vi "StateShooter.vi"(1 "Master State":enum16{"Normal", "Climb"}(ring)) -> (0 "Shooter Firing":bool)   [LabVIEW 2020]
doc: "Performs all of the calculations and decisions related to the shooter including the cowl positon."
uses:
  3e13d083-b44f-41ac-8210-6ef27915361f.vi
  31b76865-9f3e-4ec7-bf23-6a72130b3556.vi
  drivercommands.vi
  robotoutputs.vi
  robotconstants.vi
  driverdata.vi
  autonomousinfo.vi
  sensordata.vi
panel:
  in  "Max Robot Velocity Change (ft/s)":dbl=0.5
  in  "Kicker Goal Speed (rpm)":dbl=3000.0
  in  "Acceptable Kicker Error (rpm)":dbl=150.0
  in  "Acceptable Upper Shooter Error (rpm)":dbl=250.0
  in  "Minimum Range (in)":dbl=50.0
  in  "Maximum Range (in)":dbl=300.0
  in  "Acceptable Cowl Error (deg)":dbl=1.0
  in  "Acceptable Lower Shooter Error (rpm)":dbl=150.0
  in  "Settling Time (ms)":u32=100
  in  "Shooter Prespin (ms)":u32=30000
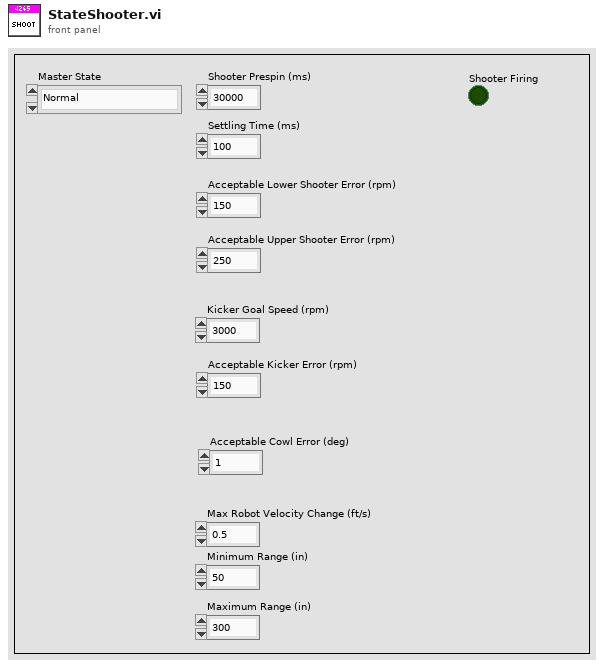
[diagram p1: front panel]
types:
  T1 = enum16{"Targetting Computer", "Position 1", "Position 2", "Position 3", "Position 4"}
  T2 = typedef "WPI_DriverStationAllianceInfo.ctl" = enum16{"Red", "Blue", "Invalid"}
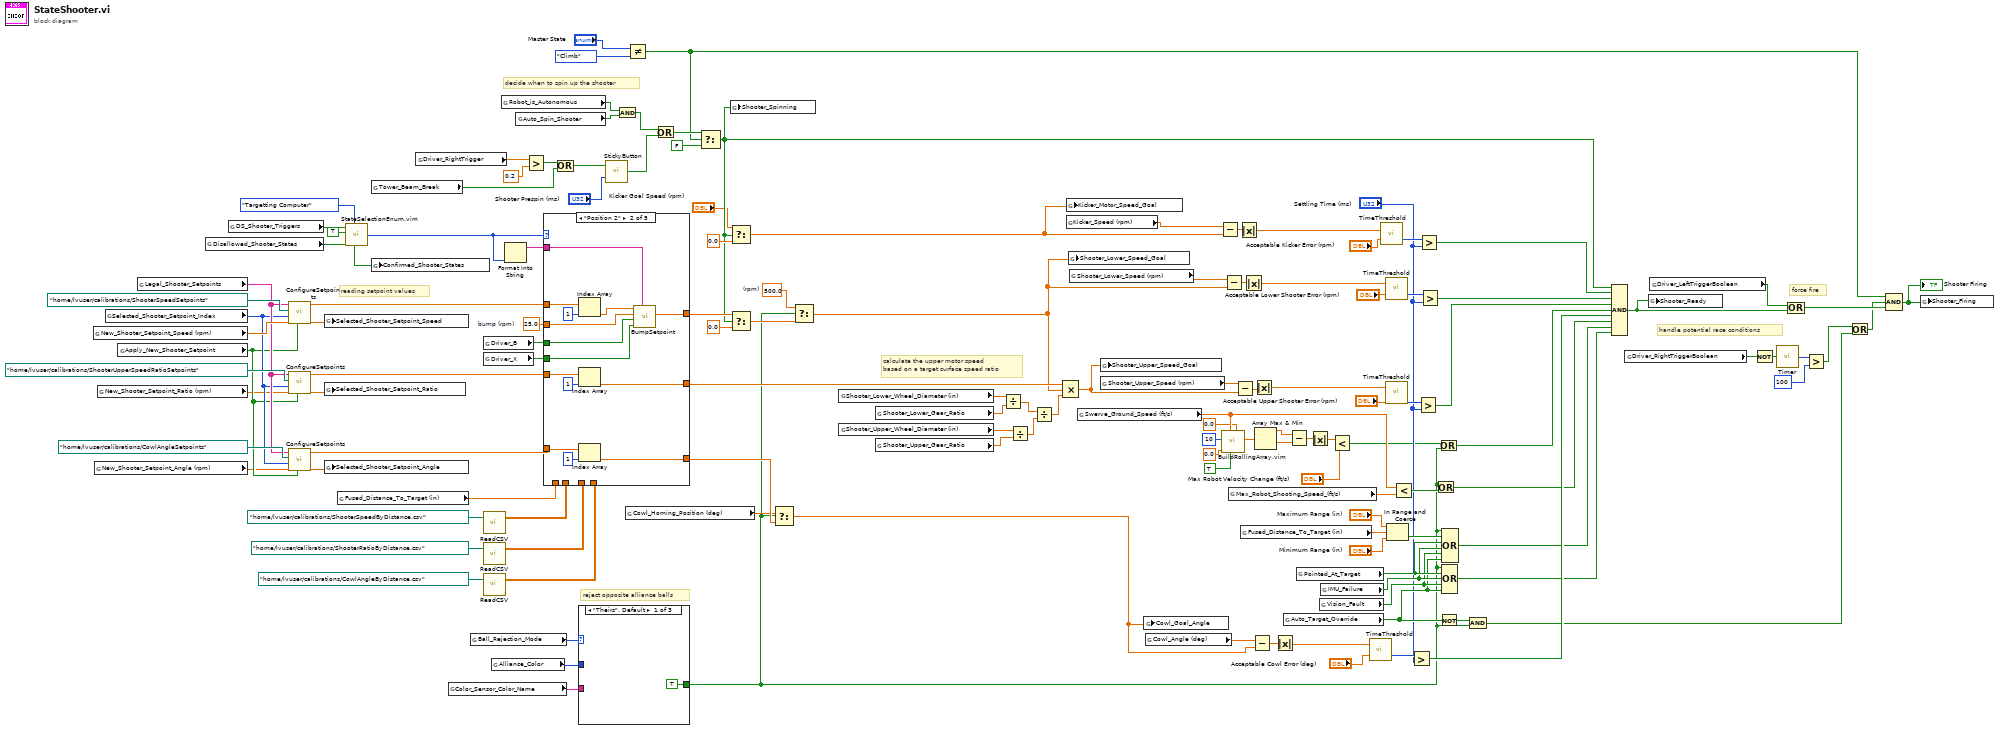
[diagram p0: block diagram]
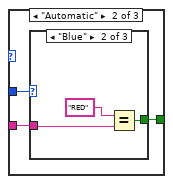
[diagram p2: hidden frame]
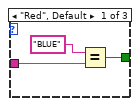
[diagram p3: hidden frame]
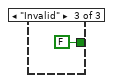
[diagram p4: hidden frame]
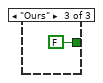
[diagram p5: hidden frame]
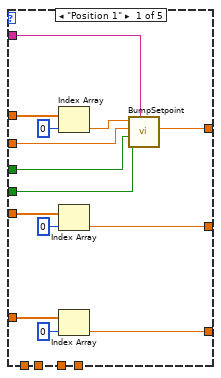
[diagram p6: hidden frame]
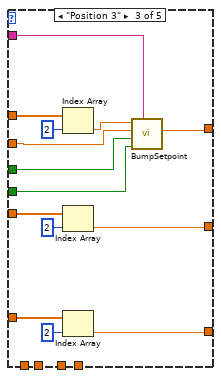
[diagram p7: hidden frame]
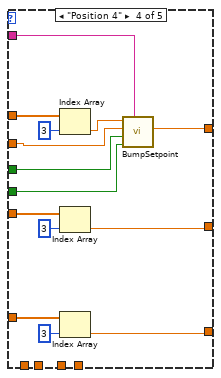
[diagram p8: hidden frame]
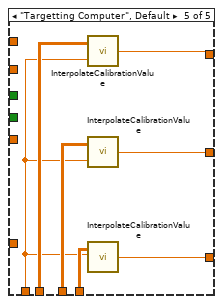
[diagram p9: hidden frame]
diagram:
  w1 = 500.0  # (rpm)
  w84 = 25.0  # bump (rpm)
  # "handle potential race conditions"
  # "calculate the upper motor speed\nbased on a target surface speed ratio"
  # "reject opposite alliance balls"
  # "force fire"
  # "reading setpoint values"
  # "decide when to spin up the shooter"
  n1 = global read "driverdata.vi" "New_Shooter_Setpoint_Speed (rpm)"() -> (w129:dbl)
  n2 = global read "driverdata.vi" "New_Shooter_Setpoint_Angle (rpm)"() -> (w119:dbl)
  n3 = global read "driverdata.vi" "New_Shooter_Setpoint_Ratio (rpm)"() -> (w120:dbl)
  n4 = global read "driverdata.vi" "Selected_Shooter_Setpoint_Index"() -> (w123:i32)
  n5 = global read "driverdata.vi" "Apply_New_Shooter_Setpoint"() -> (w121:bool)
  n6 = global read "robotconstants.vi" "Legal_Shooter_Setpoints"() -> (w124:string[])
  n7 = global read "robotoutputs.vi" "Disallowed_Shooter_States"() -> (w133:bool[])
  n8 = global read "drivercommands.vi" "DS_Shooter_Triggers"() -> (w135:bool[])
  n9 = call "ConfigureSetpoints.vi"("Apply New Setpoint"=w121, "New Setpoint"=w129, "Selected Setpoint Index"=w123, "Setpoint Save Location"=path "/home/lvuser/calibrations/ShooterSpeedSetpoints", "Setpoint Names"=w124) -> ("Selected Setpoint Value"=w118:dbl, "Setpoints"=w128:dbl[])  [unwired: 5 in]
  n10 = call "ConfigureSetpoints.vi"("Apply New Setpoint"=w121, "New Setpoint"=w120, "Selected Setpoint Index"=w123, "Setpoint Save Location"=path "/home/lvuser/calibrations/ShooterUpperSpeedRatioSetpoints", "Setpoint Names"=w124) -> ("Selected Setpoint Value"=w117:dbl, "Setpoints"=w126:dbl[])  [unwired: 5 in]
  n11 = call "ConfigureSetpoints.vi"("Apply New Setpoint"=w121, "New Setpoint"=w119, "Selected Setpoint Index"=w123, "Setpoint Save Location"=path "/home/lvuser/calibrations/CowlAngleSetpoints", "Setpoint Names"=w124) -> ("Selected Setpoint Value"=w116:dbl, "Setpoints"=w122:dbl[])  [unwired: 5 in]
  n12 = global write "robotoutputs.vi" "Selected_Shooter_Setpoint_Speed"(w118) -> ()
  n13 = global write "robotoutputs.vi" "Selected_Shooter_Setpoint_Ratio"(w117) -> ()
  n14 = global write "robotoutputs.vi" "Selected_Shooter_Setpoint_Angle"(w116) -> ()
  n15 = global read "sensordata.vi" "Fused_Distance_To_Target (in)"() -> (w87:dbl)
  n16 = call "StateSelectionEnum.vim"("Enum Def"=T1."Targetting Computer", "Disallowed States"=w133, "Enable Edge Trigger"=TRUE, "State Triggers"=w135) -> ("Selected State"=w81:T1, "Confirmed States"=w132:bool[])  [unwired: 1 in]
  n17 = global read "sensordata.vi" "Tower_Beam_Break"() -> (w41:bool)
  n18 = global write "robotoutputs.vi" "Confirmed_Shooter_States"(w132) -> ()
  n19 = global read "drivercommands.vi" "Driver_RightTrigger"() -> (w113:dbl)
  n20 = global read "sensordata.vi" "Color_Sensor_Color_Name"() -> (w64:string)
  n21 = global read "driverdata.vi" "Ball_Rejection_Mode"() -> (w61:enum16{"Theirs", "Automatic", "Ours"})
  n22 = call "ReadCSV.vi"("File Path (.csv)"=path "/home/lvuser/calibrations/ShooterSpeedByDistance.csv" ("Setpoint Save Location")) -> ("Data (index by row)"=w88:dbl[][])  [unwired: 1 in, 1 out]
  n23 = call "ReadCSV.vi"("File Path (.csv)"=path "/home/lvuser/calibrations/ShooterRatioByDistance.csv" ("Setpoint Save Location")) -> ("Data (index by row)"=w86:dbl[][])  [unwired: 1 in, 1 out]
  n24 = call "ReadCSV.vi"("File Path (.csv)"=path "/home/lvuser/calibrations/CowlAngleByDistance.csv" ("Setpoint Save Location")) -> ("Data (index by row)"=w85:dbl[][])  [unwired: 1 in, 1 out]
  n25 = global read "drivercommands.vi" "Driver_B"() -> (w83:bool)
  n26 = global read "drivercommands.vi" "Driver_X"() -> (w82:bool)
  n27 = global read "driverdata.vi" "Alliance_Color"() -> (w65:T2)
  n28 = global read "driverdata.vi" "Robot_is_Autonomous"() -> (w106:bool)
  n29 = Format Into String(w81) -> (resulting string=w80:string)  [unwired: 3 in, 1 out]
  n30 = global read "autonomousinfo.vi" "Auto_Spin_Shooter"() -> (w107:bool)
  n31 = Greater?(x=w113, y=0.2) -> (0:w111:bool)
  n32 = case shown="\"Position 2\"" w81 {
    tunnel: w128 -> [w149 w160 w174 w188 _]
    tunnel: w126 -> [w146 w159 w173 w187 _]
    tunnel: w122 -> [w143 w158 w172 w186 _]
    tunnel: [w137 w150 w168 w183 w197] -> w115
    tunnel: [w145 w157 w171 w185 w195] -> w45
    tunnel: [w142 w156 w170 w184 w192] -> w63
    tunnel: w88 -> [_ _ _ _ w198]
    tunnel: w87 -> [_ _ _ _ w193]
    tunnel: w86 -> [_ _ _ _ w196]
    tunnel: w85 -> [_ _ _ _ w194]
    tunnel: w84 -> [w140 w154 w166 w180 _]
    tunnel: w83 -> [w139 w153 w165 w179 _]
    tunnel: w82 -> [w138 w152 w164 w178 _]
    tunnel: w80 -> [w136 w151 w167 w181 _]
    frame "Position 1" {
      n33 = Index Array(array=w149, index=0) -> (element=w141:dbl)
      n34 = Index Array(array=w146, index=0) -> (element=w145:dbl)
      n35 = Index Array(array=w143, index=0) -> (element=w142:dbl)
      n36 = call "BumpSetpoint.vi"("Setpoint Name"=w136, "Bump Down Trigger"=w138, "Bump Up Trigger"=w139, "Bump Increment"=w140, "Original Setpoint"=w141) -> ("Bumped Setpoint"=w137:dbl)  [unwired: 6 in]
    }
    frame "Position 2" {
      n37 = Index Array(array=w160, index=1) -> (element=w155:dbl)
      n38 = Index Array(array=w159, index=1) -> (element=w157:dbl)
      n39 = Index Array(array=w158, index=1) -> (element=w156:dbl)
      n40 = call "BumpSetpoint.vi"("Setpoint Name"=w151, "Bump Down Trigger"=w152, "Bump Up Trigger"=w153, "Bump Increment"=w154, "Original Setpoint"=w155) -> ("Bumped Setpoint"=w150:dbl)  [unwired: 6 in]
    }
    frame "Position 3" {
      n41 = Index Array(array=w174, index=2) -> (element=w169:dbl)
      n42 = Index Array(array=w173, index=2) -> (element=w171:dbl)
      n43 = Index Array(array=w172, index=2) -> (element=w170:dbl)
      n44 = call "BumpSetpoint.vi"("Setpoint Name"=w167, "Bump Down Trigger"=w164, "Bump Up Trigger"=w165, "Bump Increment"=w166, "Original Setpoint"=w169) -> ("Bumped Setpoint"=w168:dbl)  [unwired: 6 in]
    }
    frame "Position 4" {
      n45 = Index Array(array=w188, index=3) -> (element=w182:dbl)
      n46 = Index Array(array=w187, index=3) -> (element=w185:dbl)
      n47 = Index Array(array=w186, index=3) -> (element=w184:dbl)
      n48 = call "BumpSetpoint.vi"("Setpoint Name"=w181, "Bump Down Trigger"=w178, "Bump Up Trigger"=w179, "Bump Increment"=w180, "Original Setpoint"=w182) -> ("Bumped Setpoint"=w183:dbl)  [unwired: 6 in]
    }
    frame "Targetting Computer", Default {
      n49 = call "InterpolateCalibrationValue.vi"("Input"=w193, "Calibration Data"=w198) -> ("Interpolated Output"=w197:dbl)
      n50 = call "InterpolateCalibrationValue.vi"("Input"=w193, "Calibration Data"=w196) -> ("Interpolated Output"=w195:dbl)
      n51 = call "InterpolateCalibrationValue.vi"("Input"=w193, "Calibration Data"=w194) -> ("Interpolated Output"=w192:dbl)
    }
  }
  n52 = Compound Arithmetic op=OR(w111, w41) -> (w110:bool)
  n53 = case shown="\"Theirs\", Default" w61 {
    tunnel: w65 -> [_ w202 _]
    tunnel: w64 -> [_ w201 _]
    tunnel: [TRUE w200 FALSE] -> w2
    frame "Theirs", Default {
    }
    frame "Automatic" {
      n54 = case shown="\"Blue\"" w202 {
        tunnel: w201 -> [w205 w207 _]
        tunnel: [w203 w206 FALSE] -> w200
        frame "Red", Default {
          n55 = Equal?(x="BLUE", y=w205) -> (x = y?=w203:bool)
        }
        frame "Blue" {
          n56 = Equal?(x="RED", y=w207) -> (x = y?=w206:bool)
        }
        frame "Invalid" {
        }
      }
    }
    frame "Ours" {
    }
  }
  n57 = call "StickyButton.vi"("Time threshold (ms)"="Shooter Prespin (ms)", "Button Input"=w110) -> ("Sticky Button"=w104:bool)
  n58 = And(x=w106, y=w107) -> (x .and. y?=w105:bool)
  n59 = global read "robotconstants.vi" "Cowl_Homing_Position (deg)"() -> (w52:dbl)
  n60 = Not Equal?(x="Master State", y=enum16{"Normal", "Climb"}."Climb" ("Master State")) -> (x != y?=w93:bool)
  n61 = Or(x=w105, y=w104) -> (x .or. y?=w103:bool)
  n62 = Select(t=w103, s=w93, f=FALSE) -> (s? t:f=w21:bool)
  n63 = global write "robotoutputs.vi" "Shooter_Spinning"(w21) -> ()
  n64 = Select(t="Kicker Goal Speed (rpm)", s=w21, f=0.0) -> (s? t:f=w25:dbl)
  n65 = Select(t=w115, s=w21, f=0.0) -> (s? t:f=w4:dbl)
  n66 = Select(t=w52, s=w2, f=w63) -> (s? t:f=w62:dbl)
  n67 = Select(t=w1, s=w2, f=w4) -> (s? t:f=w3:dbl)
  n68 = global read "robotconstants.vi" "Shooter_Lower_Wheel_Diameter (in)"() -> (w59:dbl)
  n69 = global read "robotconstants.vi" "Shooter_Upper_Wheel_Diameter (in)"() -> (w56:dbl)
  n70 = global read "robotconstants.vi" "Shooter_Lower_Gear_Ratio"() -> (w58:dbl)
  n71 = global read "robotconstants.vi" "Shooter_Upper_Gear_Ratio"() -> (w55:dbl)
  n72 = Divide(x=w59, y=w58) -> (x/y=w57:dbl)
  n73 = Divide(x=w56, y=w55) -> (x/y=w54:dbl)
  n74 = Divide(x=w57, y=w54) -> (x/y=w53:dbl)
  n75 = Compound Arithmetic op=MULTIPLY(w45, w3, w53) -> (w39:dbl)
  n76 = global read "sensordata.vi" "Kicker_Speed (rpm)"() -> (w26:dbl)
  n77 = global write "robotoutputs.vi" "Kicker_Motor_Speed_Goal"(w25) -> ()
  n78 = global write "robotoutputs.vi" "Shooter_Lower_Speed_Goal"(w3) -> ()
  n79 = global read "sensordata.vi" "Shooter_Lower_Speed (rpm)"() -> (w79:dbl)
  n80 = global read "sensordata.vi" "Swerve_Ground_Speed (ft/s)"() -> (w17:dbl)
  n81 = global write "robotoutputs.vi" "Shooter_Upper_Speed_Goal"(w39) -> ()
  n82 = global read "sensordata.vi" "Shooter_Upper_Speed (rpm)"() -> (w40:dbl)
  n83 = global write "robotoutputs.vi" "Cowl_Goal_Angle"(w62) -> ()
  n84 = global read "sensordata.vi" "Cowl_Angle (deg)"() -> (w73:dbl)
  n85 = Subtract(x=w26, y=w25) -> (x-y=w27:dbl)
  n86 = call "BuildRollingArray.vim"("Global Additive Update"=0.0, "Update?"=TRUE, "New Value"=w17, "Initial Value"=0.0, "Number of Elements"=10) -> ("Current Array"=w12:dbl[])  [unwired: 6 in]
  n87 = Subtract(x=w79, y=w3) -> (x-y=w101:dbl)
  n88 = global read "robotconstants.vi" "Max_Robot_Shooting_Speed_(ft/s)"() -> (w38:dbl)
  n89 = Subtract(x=w40, y=w39) -> (x-y=w100:dbl)
  n90 = Absolute Value(x=w27) -> (abs(x)=w24:dbl)
  n91 = global read "sensordata.vi" "Fused_Distance_To_Target (in)"() -> (w68:dbl)
  n92 = Absolute Value(x=w101) -> (abs(x)=w78:dbl)
  n93 = Subtract(x=w73, y=w62) -> (x-y=w99:dbl)
  n94 = Absolute Value(x=w100) -> (abs(x)=w77:dbl)
  n95 = Array Max & Min(array=w12) -> (max value=w11:dbl, min value=w10:dbl)  [unwired: 2 out]
  n96 = Absolute Value(x=w99) -> (abs(x)=w96:dbl)
  n97 = global read "driverdata.vi" "Auto_Target_Override"() -> (w36:bool)
  n98 = Subtract(x=w11, y=w10) -> (x-y=w9:dbl)
  n99 = global read "sensordata.vi" "Pointed_At_Target"() -> (w44:bool)
  n100 = Absolute Value(x=w9) -> (abs(x)=w8:dbl)
  n101 = global read "sensordata.vi" "Vision_Fault"() -> (w42:bool)
  n102 = global read "sensordata.vi" "IMU_Failure"() -> (w43:bool)
  n103 = Less?(x=w8, y="Max Robot Velocity Change (ft/s)") -> (x < y?=w7:bool)
  n104 = call "TimeThreshold.vi"("Threshold"="Acceptable Cowl Error (deg)", "Current Value"=w96) -> ("Time Below Threshold (ms)"=w60:u32)  [unwired: 1 out]
  n105 = call "TimeThreshold.vi"("Threshold"="Acceptable Kicker Error (rpm)", "Current Value"=w24) -> ("Time Below Threshold (ms)"=w23:u32)  [unwired: 1 out]
  n106 = call "TimeThreshold.vi"("Threshold"="Acceptable Lower Shooter Error (rpm)", "Current Value"=w78) -> ("Time Below Threshold (ms)"=w75:u32)  [unwired: 1 out]
  n107 = call "TimeThreshold.vi"("Threshold"="Acceptable Upper Shooter Error (rpm)", "Current Value"=w77) -> ("Time Below Threshold (ms)"=w74:u32)  [unwired: 1 out]
  n108 = In Range and Coerce(upper limit="Maximum Range (in)", x=w68, lower limit="Minimum Range (in)") -> (In Range?=w49:bool)  [unwired: 1 out]
  n109 = Less?(x=w17, y=w38) -> (x < y?=w50:bool)
  n110 = Greater?(x=w60, y="Settling Time (ms)") -> (0:w95:bool)
  n111 = Greater?(x=w74, y="Settling Time (ms)") -> (0:w97:bool)
  n112 = Greater?(x=w23, y="Settling Time (ms)") -> (0:w20:bool)
  n113 = Greater?(x=w75, y="Settling Time (ms)") -> (0:w98:bool)
  n114 = Or(x=w2, y=w50) -> (x .or. y?=w51:bool)
  n115 = Or(x=w7, y=w2) -> (x .or. y?=w6:bool)
  n116 = Not(x=w36) -> (.not. x?=w35:bool)
  n117 = Compound Arithmetic op=OR(w2, w44, w43, w42, w36) -> (w47:bool)
  n118 = Compound Arithmetic op=OR(w2, w49, w44, w43, w42, w36) -> (w48:bool)
  n119 = And(x=w35, y=w2) -> (x .and. y?=w34:bool)
  n120 = Compound Arithmetic op=AND(w21, w20, w98, w97, w6, w95, w51, w48, w47) -> (w71:bool)
  n121 = global read "drivercommands.vi" "Driver_RightTriggerBoolean"() -> (w33:bool)
  n122 = global write "robotoutputs.vi" "Shooter_Ready"(w71) -> ()
  n123 = global read "drivercommands.vi" "Driver_LeftTriggerBoolean"() -> (w70:bool)
  n124 = Not(x=w33) -> (.not. x?=w32:bool)
  n125 = call "Timer.vi"("Reset Timer"=w32) -> ("Time (ms)"=w31:u32)
  n126 = Compound Arithmetic op=OR(w70, w71) -> (w69:bool)
  n127 = Greater?(x=w31, y=u32 100) -> (0:w29:bool)
  n128 = Or(x=w29, y=w34) -> (x .or. y?=w37:bool)
  n129 = Compound Arithmetic op=AND(w93, w37, w69) -> (w92:bool)
  "Shooter Firing" <- w92
  n130 = global write "robotoutputs.vi" "Shooter_Firing"(w92) -> ()
